vi "Send Case-Controller.vi"(5 "Message Type":refnum<class "Case-Controller Msg.lvclass">, 7 "Message Priority (Normal)":T1=enum."Normal", 8 "error in (no error)":errorcluster, 10 "Controller Case":string, 11 "Message Enqueuer":refnum<class "Message Enqueuer.lvclass">) -> (0 "error out":errorcluster, 3 "Message Enqueuer out":refnum<class "Message Enqueuer.lvclass">)   [LabVIEW 2025, in "UserConsole.lvlib" / "Case-Controller Msg.lvclass"]
doc: "This VI sends the message to an actor."
uses:
  Case-Controller Msg.lvclass
  <vilib>/ActorFramework/Message Enqueuer/Message Enqueuer.lvclass
  <vilib>/ActorFramework/Message Enqueuer/Message Priority.ctl
  C:/Program Files (x86)/National Instruments/LabVIEW 2025/vi.lib/ActorFramework/Message/Message.lvclass
  Case-Controller Msg.lvclass/Case-Controller Msg.ctl
  <vilib>/ActorFramework/Message Enqueuer/Message Enqueuer.lvclass/Message Enqueuer.ctl
  <vilib>/ActorFramework/Message Priority Queue/Priority Enqueue.vi
  C:/Users/halstead_rideriver/Documents/Labview_Practice/ATM_Machine_Actor Framework/ATM_ACTOR_Without_States/UserConsole Messages/Case-Controller Msg/Case-Controller Msg.lvclass
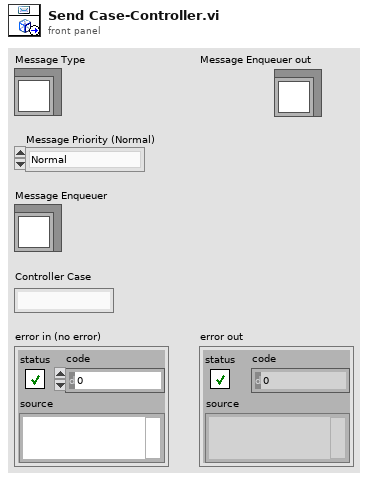
[diagram p1: front panel]
types:
  T1 = typedef "Actor Framework.lvlib/Message Enqueuer.lvclass/Message Priority.ctl" = enum16{"Low", "Normal", "High"}
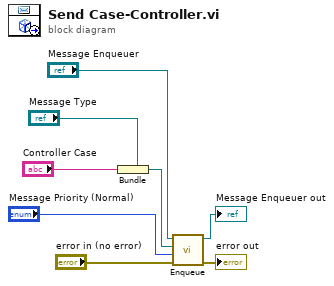
[diagram p0: block diagram]
diagram:
  n1 = Bundle(cluster="Message Type", "Controller Case") -> (w4:refnum<class "Case-Controller Msg.lvclass">)
  n2 = call <vilib>:"Enqueue.vi"("error in (no error)"="error in (no error)", "Message Priority (Normal)"="Message Priority (Normal)", "Message"=w4, "Message Enqueuer in"="Message Enqueuer") -> ("error out"=→"error out":errorcluster, "Message Enqueuer in"=→"Message Enqueuer out":refnum<class "Message Enqueuer.lvclass">)  [unwired: 6 in]
